vi "SVL RMS Level (resampled) (N Ch).vi"(6 "restart averaging (F)":bool, 8 "error in (no error)":errorcluster, 10 "even-angle channel info":T1[](array[typedef]) {"channel info"."pregain" format="%.2f"; "channel info"."weighting filter" items=["Linear", "A-weighting", "B-weighting", "C-weighting", "ITU-R 468-4", "Dolby", "CCITT", "C-message", "Wb", "Wc", "Wd", "We", "Wf", "Wh", "Wj", "Wk", "Wm", "AES17 20 kHz lowpass", "AES17 40 kHz lowpass", "AES17 20 kHz highpass", "AES17 40 kHz highpass"]; "channel info"."dB reference" format="%^.1e"; "channel info"."engineering units" items=["custom..."=0, "V"=1, "A"=21, "C"=30, "pC"=31, "s"=32, "-"=29, "Pa"=2, "N"=20, "g"=3, "m/s^2"=4, "m/s"=5, "m"=6, "mm/s"=12, "mm"=13, "micron/s"=14, "micron"=15, "in/s^2"=7, "in/s"=8, "in"=9, "mil/s"=10, "mil"=11, "rad/s^2"=16, "rad/s"=17, "rad"=18, "deg/s^2"=26, "deg/s"=27, "deg"=28, "RPM"=22, "cycle/s^2"=23, "Hz"=24, "cycle"=25, "strain"=19]; "channel info"."sensor sensitivity" format="%#_5f"}, 11 "even-angle signals [EU]":T5(array[cluster]) {"even-angle signal" format="%.2f"; "dr" format="%.2f"; "r0" format="%.2f"}) -> (0 "error out":errorcluster, 2 "unit labels":string[](array[string]), 3 "RMS levels [EU rms]":dbl[](array[numeric]) format="%.2f")   [LabVIEW 2017, in "SoundVib_VibrationLevel.lvlib"]
doc: "Computes the root-mean-square (RMS) level of <B>scaled signal [EU]</B> or <B>even-angle signal [EU]</B>. <B>Scaled signal [EU]</B> should have a zero DC component. You can attenuate the DC component with hardware AC-coupling filters and with software high-pass filters. Wire data to the <B>scaled signal [EU]</B> input to determine the polymorphic instance to use or manually select the instance."
uses:
  <vilib>/addons/Sound and Vibration/svt_Level/SoundVib_VibrationLevel.lvlib
  <vilib>/addons/_NISVFA/_Shared subVIs/Controls/svc_Resampled Channel Info.ctl
  <vilib>/addons/_NISVFA/_Shared subVIs/Controls/svc_Channel Info.ctl
  <vilib>/addons/_NISVFA/_Shared subVIs/Controls/svc_Engineering Units Text Ring.ctl
  <vilib>/addons/_NISVFA/_Shared subVIs/Controls/svc_Weighting Filter Text Ring.ctl
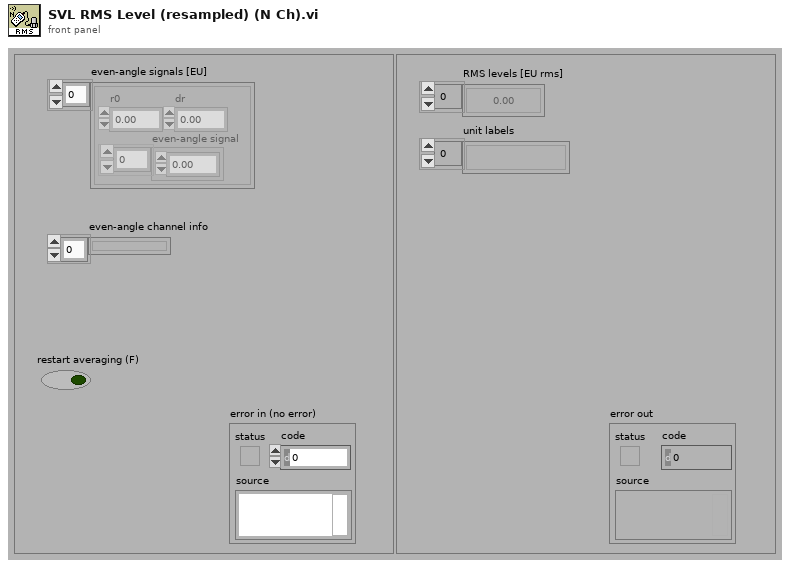
[diagram p1: front panel]
types:
  T1 = typedef "svc_Resampled Channel Info.ctl" = cluster{"channel name":string, "description":string, " channel info":T2}
  T2 = typedef "svc_Channel Info.ctl" = cluster{"sensor sensitivity":dbl, "engineering units":T3, "dB reference":dbl, "custom label":string, "weighting filter":T4, "pregain":dbl}
  T3 = typedef "svc_Engineering Units Text Ring.ctl" = u16
  T4 = typedef "svc_Weighting Filter Text Ring.ctl" = u16
  T5 = cluster{"r0":dbl, "dr":dbl, "even-angle signal":dbl[]}[]
  T6 = enum16{"RMS", "Running RMS", "Exp avg  ", "Dec exp avg ", "Peak", "Crest"}
  T7 = cluster{"r0":dbl, "dr":dbl, "even angle signal":dbl[]}[]
  T8 = enum16{"Reset filter", "Restart averaging", "Continue processing"}
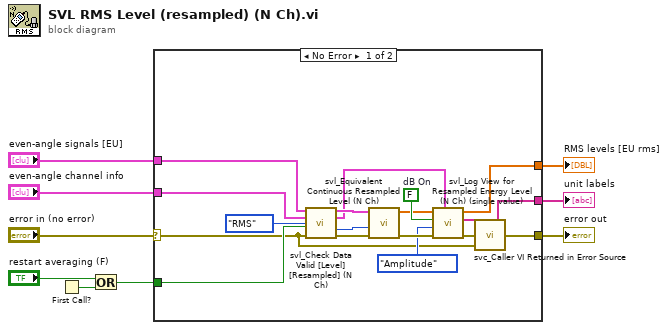
[diagram p0: block diagram]
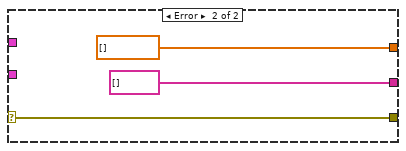
[diagram p2: hidden frame]
diagram:
  n1 = First Call?() -> (First Call?: T/F=w5:bool)
  n2 = Or(x="restart averaging (F)", y=w5) -> (x .or. y?=w3:bool)
  n3 = case shown="No Error" "error in (no error)" {
    selector: "error in (no error)" -> [w10 w29]
    tunnel: [w19 w29] -> w9
    tunnel: [w22 dbl[] [] ("energy levels [EU^2 rms]")] -> w8
    tunnel: [w21 string[] [] ("unit label [ ]")] -> w7
    tunnel: "even-angle signals [EU]" -> [w13 _]
    tunnel: w3 -> [w16 _]
    tunnel: "even-angle channel info" -> [w12 _]
    frame No Error {
      w24 = FALSE  # dB On
      n4 = call <vilib>:"svl_Check Data Valid [Level] [Resampled] (N Ch).vi"("scaled even angle signals [EU]"=w13, "even angle channel info"=w12, "level analysis"=T6."RMS" ("Level Analysis"), "restart averaging (F)"=w16, "error in (no error)"=w10) -> ("dup scaled even angle signals [EU]"=w14:T7, "dup even angle channel info"=w11:T1[], "processing state"=w17:T8, "error out"=w18:errorcluster)  [unwired: 7 in]
      n5 = call <vilib>:"svl_Equivalent Continuous Resampled Level (N Ch).vi"("error in (no error)"=w18, "processing state"=w17, "scaled even angle signals [EU]"=w14) -> ("error out"=w25:errorcluster, "equivalent continuous levels [EU^2 rms]"=w23:dbl[])  [unwired: 7 in]
      n6 = call <vilib>:"svl_Log View for Resampled Energy Level (N Ch) (single value).vi"("even angle channel info"=w11, "error in (no error)"=w25, "view mode"=enum16{"Power", "Amplitude"}."Amplitude", "dB On (T)"=w24, "energy levels [EU^2 rms]"=w23) -> ("error out"=w26:errorcluster, "unit label [ ]"=w21:string[], "energy levels [EU^2 rms]"=w22:dbl[])  [unwired: 4 in]
      n7 = call <vilib>:"svc_Caller VI Returned in Error Source.vi"("warning input to caller"=w10, "error in (no error)"=w26) -> ("error out"=w19:errorcluster)  [unwired: 3 in]
    }
    frame Error {
    }
  }
  "RMS levels [EU rms]" <- w8
  "unit labels" <- w7
  "error out" <- w9
